vi "rad_Save Config.vi"(8 "error in (no error":errorcluster, 11 "State":T1 {"Targets Information"."Primary NIC"."IP Address Request Mode" items=["Static"=1, "DHCP/Link-Local"=2, "Link-Local Only"=4, "DHCP Only"=8]}) -> (0 "error out":errorcluster, 2 "Configuration File Path":path)   [LabVIEW 2020]
uses:
  TypeDefs/rad_State Data.ctl
  Targets/TypeDefs/rad_Targets Settings.ctl
  Targets/TypeDefs/rad_Target Information.ctl
  Targets/TypeDefs/rad_Target Network Settings.ctl
  App Images/TypeDefs/rad_App Images Settings.ctl
  App Images/TypeDefs/rad_AppImage Information.ctl
  App Images/TypeDefs/rad_Application Image Properties.ctl
  App Images/TypeDefs/rad_FPGA Properties.ctl
  App Images/TypeDefs/rad_FPGA Flash Properties.ctl
  Targets/TypeDefs/rad_Discovery Settings.ctl
  <vilib>/Utility/config.llb/Write Key (Path).vi
  rad_Globals.vi
  <vilib>/Utility/config.llb/Write Key (String).vi
  <vilib>/Utility/config.llb/Write Key (Boolean).vi
  <vilib>/Utility/config.llb/Write Key (I32).vi
  <vilib>/Utility/config.llb/Write Key (U32).vi
  <vilib>/Utility/config.llb/NI_LVConfig.lvlib
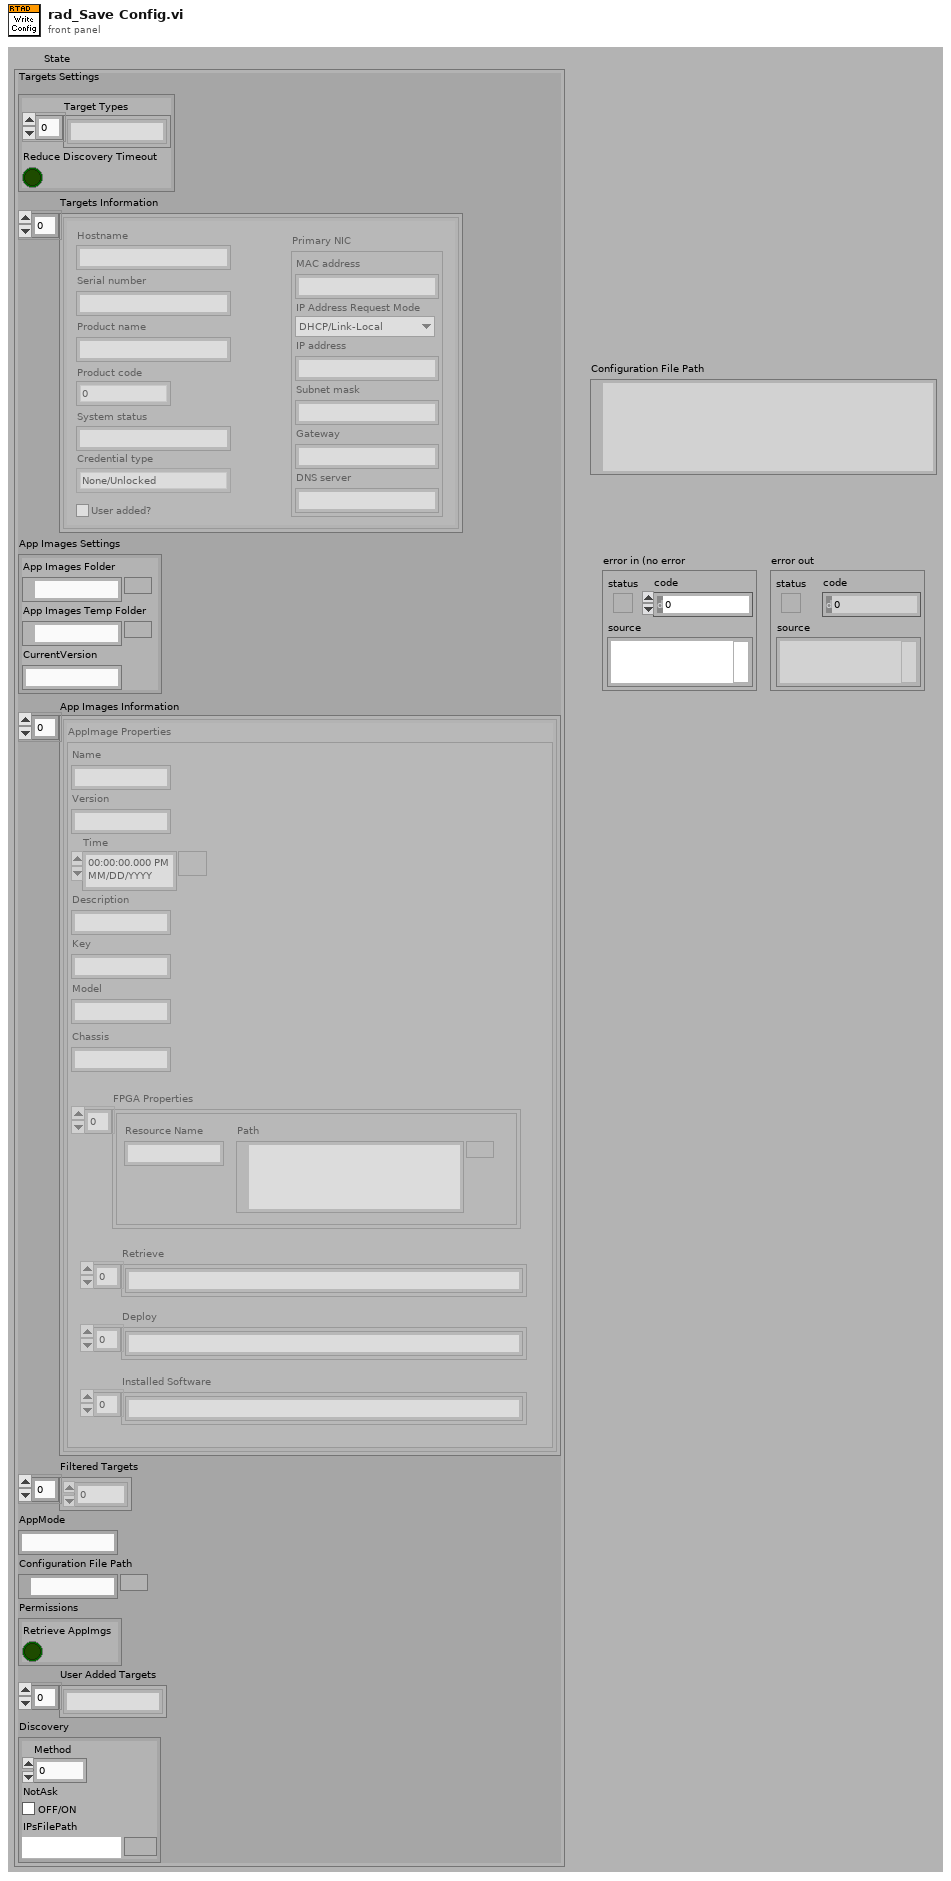
[diagram p1: front panel]
types:
  T1 = typedef "rad_State Data.ctl" = cluster{"Targets Settings":T2, "Targets Information":T3[], "App Images Settings":T5, "App Images Information":T6[], "Filtered Targets":i32[], "AppMode":string, "Configuration File Path":path, "Permissions":cluster{"Retrieve AppImgs":bool}, "User Added Targets":string[], "Discovery":T10}
  T2 = typedef "rad_Targets Settings.ctl" = cluster{"Target Types":string[], "Reduce Discovery Timeout":bool}
  T3 = typedef "rad_Target Information.ctl" = cluster{"Hostname":string, "Serial number":string, "Product name":string, "Product code":i32, "System status":string, "Credential type":enum16{"None/Unlocked", "FTP Password", "NIAuth Credentials"}, "User added?":bool, "Primary NIC":T4}
  T4 = typedef "rad_Target Network Settings.ctl" = cluster{"MAC address":string, "IP Address Request Mode":i32, "IP address":string, "Subnet mask":string, "Gateway":string, "DNS server":string}
  T5 = typedef "rad_App Images Settings.ctl" = cluster{"App Images Folder":path, "App Images Temp Folder":path, "CurrentVersion":string}
  T6 = typedef "rad_AppImage Information.ctl" = cluster{"AppImage Properties":T7, "AppImage Path":path}
  T7 = typedef "rad_Application Image Properties.ctl" = cluster{"Name":string, "Version":string, "Time":timestamp, "Description":string, "Key":string, "Chassis":string, "FPGA Properties":T8, "Model":string, "Retrieve":string[], "Deploy":string[], "Installed Software":string[]}
  T8 = typedef "rad_FPGA Properties.ctl" = T9[]
  T9 = typedef "rad_FPGA Flash Properties.ctl" = cluster{"Resource Name":string, "Path":path}
  T10 = typedef "rad_Discovery Settings.ctl" = cluster{"Method":u32, "NotAsk":bool, "IPsFilePath":path}
  T11 = typedef "NI_LVConfig.lvlib/Config Data RefNum.ctl" = refnum<k1>
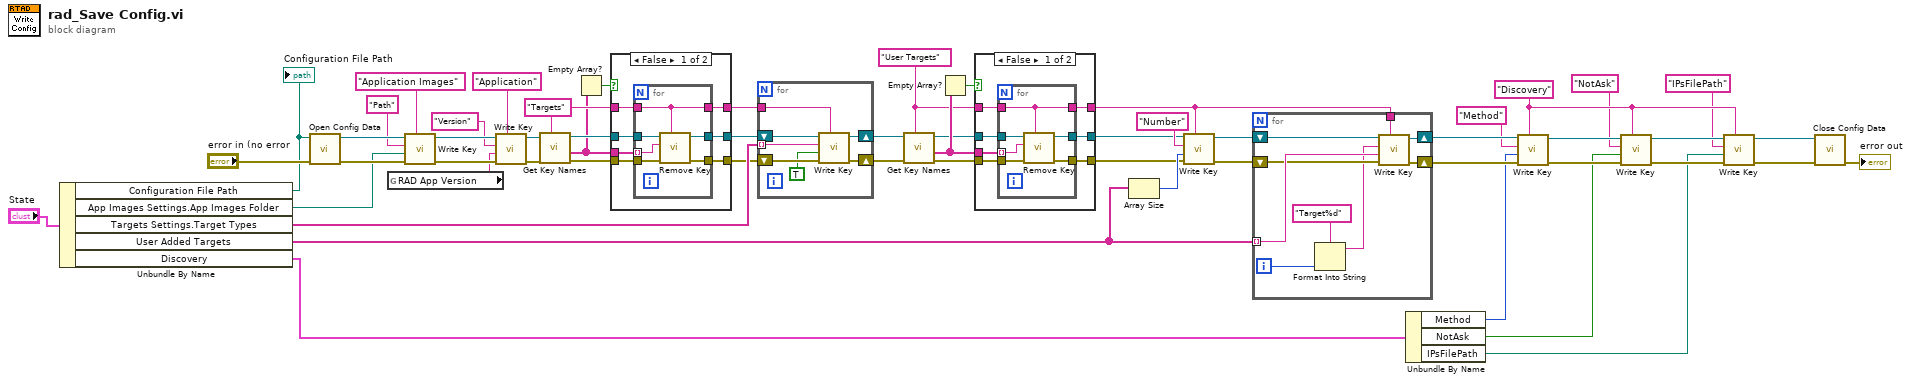
[diagram p0: block diagram]
diagram:
  w8 = "Discovery" ("section")
  w26 = "User Targets" ("section")
  w50 = "Targets" ("section")
  n1 = Unbundle By Name("State") -> ("Configuration File Path"=w16:path, "App Images Settings.App Images Folder"=w52:path, "Targets Settings.Target Types"=w49:string[], "User Added Targets"=w25:string[], "Discovery"=w4:T10)
  "Configuration File Path" <- w16
  n2 = call <vilib>:"Open Config Data.vi"("error in (no error)"="error in (no error", "configuration file path"=w16) -> ("error out"=w55:errorcluster, "refnum"=w54:T11)  [unwired: 7 in, 1 out]
  n3 = global read "rad_Globals.vi" "RAD App Version"() -> (w18:string)
  n4 = call-poly <vilib>:"Write Key.vi"("section"="Application Images", "error in (no error)"=w55, "value"=w52, "key"="Path", "refnum"=w54) -> ("error out"=w23:errorcluster, "refnum out"=w24:T11)  [unwired: 1 in, 4 out]
  n5 = call-poly <vilib>:"Write Key.vi"("section"="Application", "error in (no error)"=w23, "value"=w18, "key"="Version", "refnum"=w24) -> ("error out"=w19:errorcluster, "refnum out"=w20:T11)  [unwired: 1 in, 4 out]
  n6 = call <vilib>:"Get Key Names.vi"("section"=w50, "error in (no error)"=w19, "refnum"=w20) -> ("error out"=w51:errorcluster, "key names"=w45:string[], "refnum out"=w46:T11)  [unwired: 6 out]
  n7 = Empty Array?(array=w45) -> (empty?=w44:bool)
  n8 = case shown="False" w44 {
    tunnel: w51 -> [w63 w70]
    tunnel: w45 -> [w62 _]
    tunnel: w50 -> [w61 w72]
    tunnel: w46 -> [w60 w71]
    tunnel: [w57 w72] -> w43
    tunnel: [w59 w71] -> w42
    tunnel: [w58 w70] -> w41
    frame False {
      n9 = for {
        tunnel: w63 -> [w69]
        tunnel: w60 -> [w66]
        tunnel: w62 -> [w67] mode=indexing
        tunnel: w61 -> [w68]
        tunnel: [w68] -> w57
        tunnel: [w65] -> w58
        tunnel: [w64] -> w59
        n10 = call <vilib>:"Remove Key.vi"("section"=w68, "error in (no error)"=w69, "key"=w67, "refnum"=w66) -> ("error out"=w65:errorcluster, "refnum out"=w64:T11)  [unwired: 6 out]
      }
    }
    frame True {
    }
  }
  n11 = for {
    tunnel: w49 -> [w76] mode=indexing
    tunnel: w43 -> [w73]
    shift-right: [w75] -> w31
    shift-left: w42 -> [w79]
    shift-right: [w74] -> w30
    shift-left: w41 -> [w78]
    n12 = call-poly <vilib>:"Write Key.vi"("section"=w73, "error in (no error)"=w78, "value"=TRUE, "key"=w76, "refnum"=w79) -> ("error out"=w74:errorcluster, "refnum out"=w75:T11)  [unwired: 1 in, 4 out]
  }
  n13 = call <vilib>:"Get Key Names.vi"("section"=w26, "error in (no error)"=w30, "refnum"=w31) -> ("error out"=w32:errorcluster, "key names"=w34:string[], "refnum out"=w33:T11)  [unwired: 6 out]
  n14 = Empty Array?(array=w34) -> (empty?=w35:bool)
  n15 = case shown="False" w35 {
    tunnel: w32 -> [w86 w93]
    tunnel: w34 -> [w85 _]
    tunnel: w26 -> [w84 w95]
    tunnel: w33 -> [w83 w94]
    tunnel: [w80 w95] -> w29
    tunnel: [w82 w94] -> w28
    tunnel: [w81 w93] -> w27
    frame False {
      n16 = for {
        tunnel: w86 -> [w92]
        tunnel: w83 -> [w89]
        tunnel: w85 -> [w90] mode=indexing
        tunnel: w84 -> [w91]
        tunnel: [w91] -> w80
        tunnel: [w88] -> w81
        tunnel: [w87] -> w82
        n17 = call <vilib>:"Remove Key.vi"("section"=w91, "error in (no error)"=w92, "key"=w90, "refnum"=w89) -> ("error out"=w88:errorcluster, "refnum out"=w87:T11)  [unwired: 6 out]
      }
    }
    frame True {
    }
  }
  n18 = Array Size(array=w25) -> (size(s)=w40:i32)
  n19 = call-poly <vilib>:"Write Key.vi"("section"=w29, "error in (no error)"=w27, "value"=w40, "key"="Number", "refnum"=w28) -> ("error out"=w37:errorcluster, "refnum out"=w38:T11)  [unwired: 1 in, 4 out]
  n20 = for {
    tunnel: w25 -> [w102] mode=indexing
    tunnel: w29 -> [w103]
    shift-right: [w100] -> w36
    shift-left: w37 -> [w101]
    shift-right: [w99] -> w13
    shift-left: w38 -> [w104]
    i -> [w97]
    n21 = Format Into String(format string="Target%d", w97) -> (resulting string=w96:string)  [unwired: 2 in, 1 out]
    n22 = call-poly <vilib>:"Write Key.vi"("section"=w103, "error in (no error)"=w101, "value"=w102, "key"=w96, "refnum"=w104) -> ("error out"=w100:errorcluster, "refnum out"=w99:T11)  [unwired: 1 in, 4 out]
  }
  n23 = Unbundle By Name(w4) -> ("Method"=w3:u32, "NotAsk"=w2:bool, "IPsFilePath"=w1:path)
  n24 = call-poly <vilib>:"Write Key.vi"("section"=w8, "error in (no error)"=w36, "value"=w3, "key"="Method", "refnum"=w13) -> ("error out"=w14:errorcluster, "refnum out"=w12:T11)  [unwired: 4 in, 1 out]
  n25 = call-poly <vilib>:"Write Key.vi"("section"=w8, "error in (no error)"=w14, "value"=w2, "key"="NotAsk", "refnum"=w12) -> ("error out"=w15:errorcluster, "refnum out"=w10:T11)  [unwired: 4 in, 1 out]
  n26 = call-poly <vilib>:"Write Key.vi"("section"=w8, "error in (no error)"=w15, "value"=w1, "key"="IPsFilePath", "refnum"=w10) -> ("error out"=w11:errorcluster, "refnum out"=w9:T11)  [unwired: 4 in, 1 out]
  n27 = call <vilib>:"Close Config Data.vi"("error in (no error)"=w11, "refnum"=w9) -> ("error out"=→"error out":errorcluster)  [unwired: 1 in, 8 out]
